vi "faux_daq.vi"() -> ()   [LabVIEW 2022 SP3]
panel:
  out "input_history":cluster{"Request":string, "Payload":variant}[](array[cluster])
  in  "clear_error":bool
  out "last output":T1
  in  "done":bool
  in  "payload":string caption="Request Payload"
  in  "request":string(combo) caption="Select Request"
  in  "send_request":bool
  in  "select_module":string(combo)="motion" caption="Select Test Module"
  out "output_history":T2(array[cluster])
  out "error out":errorcluster
  in  "error in":errorcluster
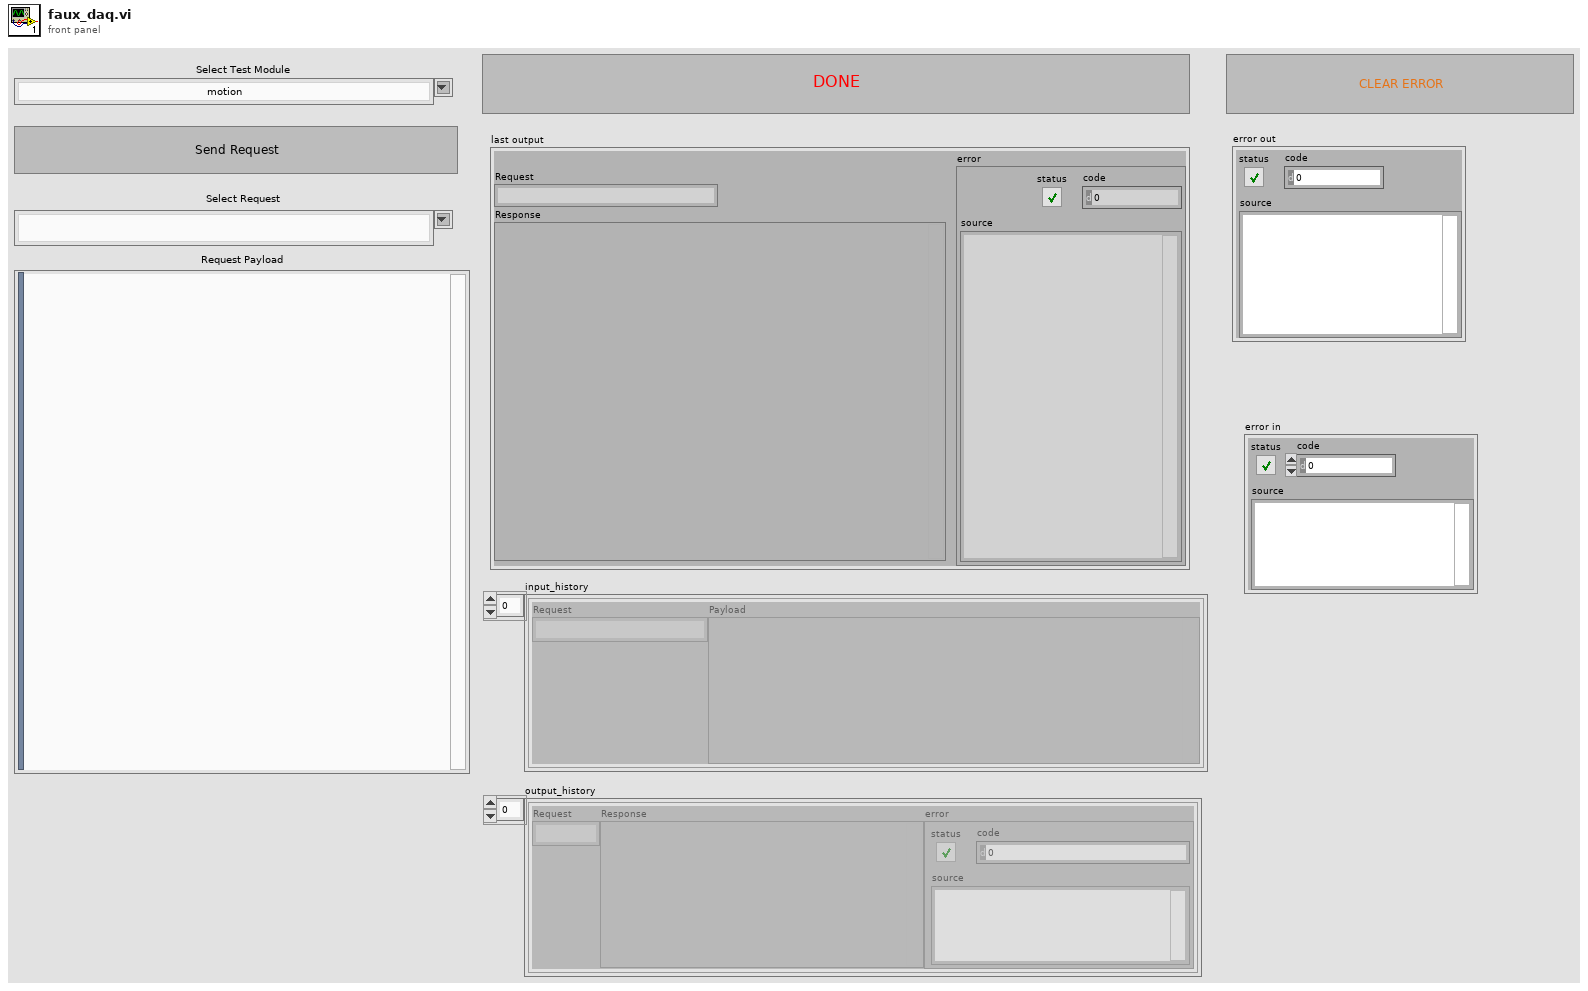
[diagram p1: front panel]
types:
  T1 = cluster{"Request":string, "Response":variant, "error":errorcluster}
  T2 = cluster{"Request":string, "Response":variant, "error":errorcluster}[]
  T3 = cluster{"request":string, "Response data":variant, "error IO":errorcluster}[]
  T4 = enum8{"Enabled", "Disabled", "Disabled and Grayed Out"}
  T5 = cluster{"request":string, "Response data":variant, "error IO":errorcluster}
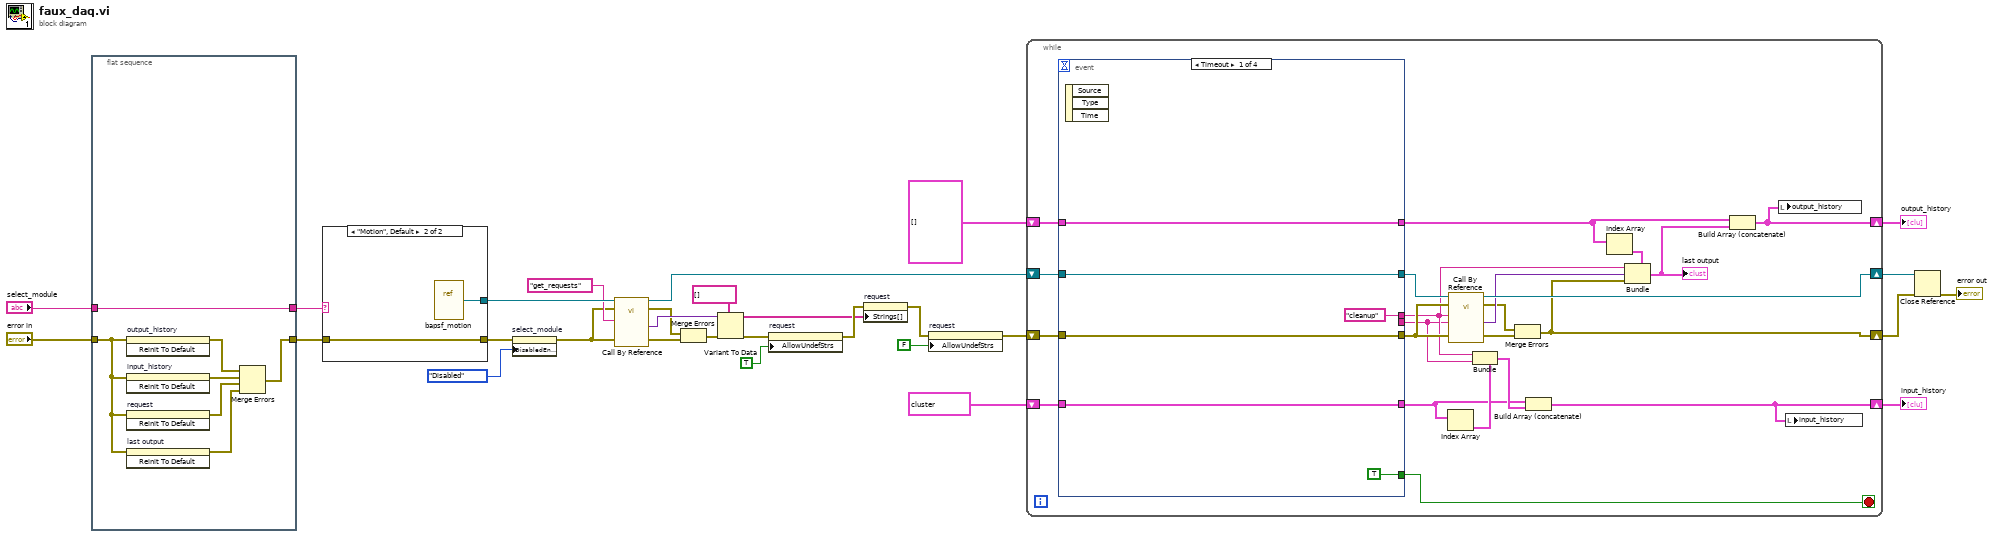
[diagram p0: block diagram]
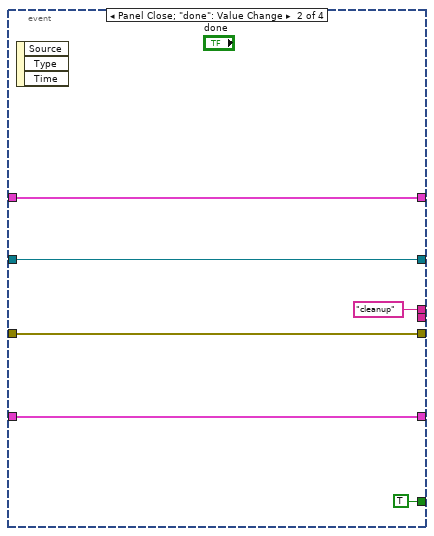
[diagram p2: hidden frame]
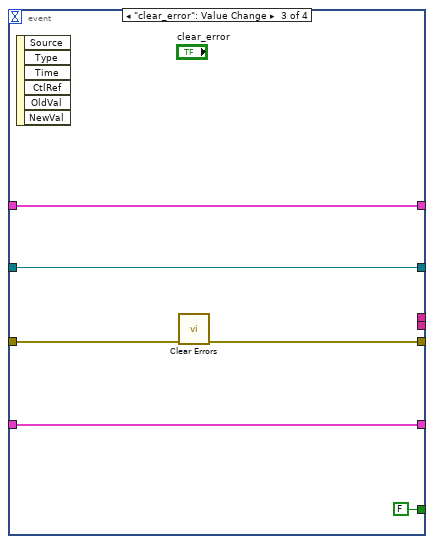
[diagram p3: hidden frame]
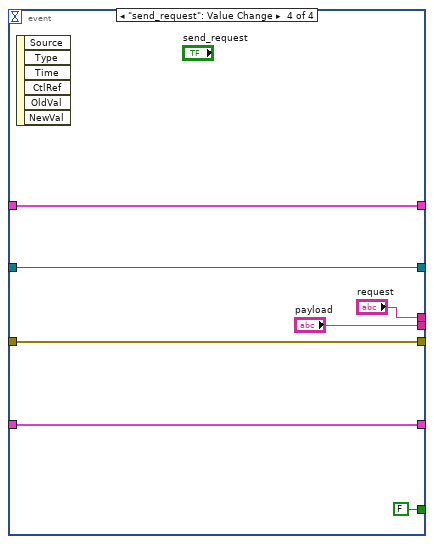
[diagram p4: hidden frame]
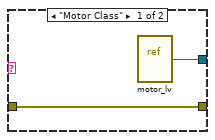
[diagram p5: hidden frame]
diagram:
  n1 = flat-sequence {
    tunnel: [w33] -> w29
    tunnel: "error in" -> [w35]
    tunnel: "select_module" -> [w36]
    tunnel: [w36] -> w5
    frame #0 {
      n2 = invoke on="output_history" class="Arr (strict)" method="Reinit To Default"(error in=w35) -> (error out=w34:errorcluster)  [unwired: 2 in, 2 out]
      n3 = invoke on="input_history" class="Arr (strict)" method="Reinit To Default"(error in=w35) -> (error out=w32:errorcluster)  [unwired: 2 in, 2 out]
      n4 = invoke on="request" class="CmbBox" method="Reinit To Default"(error in=w35) -> (error out=w31:errorcluster)  [unwired: 2 in, 2 out]
      n5 = invoke on="last output" class="Clust (strict)" method="Reinit To Default"(error in=w35) -> (error out=w30:errorcluster)  [unwired: 2 in, 2 out]
      n6 = Merge Errors(w34, w32, w31, w30) -> (w33:errorcluster)
    }
  }
  n7 = case shown="\"Motion\", Default" w5 {
    tunnel: w29 -> [w37 w39]
    tunnel: [w38 w40] -> w28
    tunnel: [w37 w39] -> w12
    frame "Motor Class" {
      n8 = vi-ref "motor_lv.vi"() -> (w38:refnum<vi>)
    }
    frame "Motion", Default {
      n9 = vi-ref "bapsf_motion.vi"() -> (w40:refnum<vi>)
    }
  }
  n10 = property on="select_module" class="CmbBox"(error in=w12, "DisabledEnum"=T4."Disabled" ("Disabled")) -> (error out=w11:errorcluster)  [unwired: 1 in, 1 out]
  n11 = call-by-ref "?"(reference=w28, error in=w11, "error in"=w11, "Request"="get_requests") -> (reference out=w15:refnum<vi>, error out=w18:errorcluster, 0:"error out"=w16:errorcluster, "Response data"=w26:variant)  [unwired: 4 in]
  n12 = Merge Errors(w18, w16) -> (w17:errorcluster)
  n13 = Variant To Data(error in=w17, type=string[] [], Variant=w26) -> (data=w21:string[], error out=w23:errorcluster)
  n14 = property on="request" class="CmbBox"(error in=w23, "AllowUndefStrs"=TRUE ("Allow Undefined Strings")) -> (error out=w22:errorcluster)  [unwired: 1 in, 1 out]
  n15 = property on="request" class="CmbBox"(error in=w22, "Strings[]"=w21) -> (error out=w20:errorcluster)  [unwired: 1 in, 1 out]
  n16 = property on="request" class="CmbBox"(error in=w20, "AllowUndefStrs"=FALSE ("Allow Undefined Strings")) -> (error out=w14:errorcluster)  [unwired: 1 in, 1 out]
  n17 = while {
    shift-right: [w58] -> w10
    shift-left: w15 -> [w60]
    shift-right: [w49] -> w9
    shift-left: w14 -> [w62]
    shift-right: [w48] -> w3
    shift-left: T3 [] -> [w56]
    shift-right: [w41] -> w1
    shift-left: cluster{"Request":string, "Payload":variant}[] [{"Request"="initialize", "Payload"=variant}, {"Request"="cleanup", "Payload"=variant}] ("input_history") -> [w47]
    stop <- w57 stop-if-true
    n18 = event shown="[0] Timeout" {
      selector: _ -> [_ _ _ _]
      dyn-events: _ -> [_ _ _ _]
      timeout: _ -> [_ _ _ _]
      tunnel: w62 -> [w68 w74 w78 w81]
      tunnel: [w68 w74 w77 w81] -> w61
      tunnel: w60 -> [w67 w70 w79 w83]
      tunnel: [w67 w70 w79 w83] -> w59
      tunnel: [TRUE TRUE FALSE FALSE] -> w57
      tunnel: ["cleanup" "cleanup" _ "request"] -> w45
      tunnel: w56 -> [w64 w71 w80 w87]
      tunnel: [w64 w71 w80 w87] -> w55
      tunnel: [_ _ _ "payload"] -> w44
      tunnel: w47 -> [w63 w69 w75 w82]
      tunnel: [w63 w69 w75 w82] -> w42
      event Timeout {
        n19 = event-data() -> ()  [unwired: 1 in, 3 out]
      }
      event Panel Close; "done": Value Change {
        n20 = event-data() -> ()  [unwired: 1 in, 3 out]
      }
      event "clear_error": Value Change {
        n21 = event-data() -> ()  [unwired: 1 in, 6 out]
        n22 = call <vilib>:"Clear Errors.vi"("error in (no error)"=w78) -> ("error out"=w77:errorcluster)  [unwired: 5 in, 1 out]
      }
      event "send_request": Value Change {
        n23 = event-data() -> ()  [unwired: 1 in, 6 out]
      }
    }
    n24 = Index Array(array=w42) -> (element=w46:cluster{"Request":string, "Payload":variant})  [unwired: 1 in]
    n25 = call-by-ref "?"(reference=w59, error in=w61, "error in"=w61, "Request data"=w44, "Request"=w45) -> (reference out=w58:refnum<vi>, error out=w51:errorcluster, 0:"error out"=w50:errorcluster, "Response data"=w52:variant)  [unwired: 3 in]
    n26 = Bundle(cluster=w46, "Request"=w45, "Payload"=w44) -> (w43:cluster{"Request":string, "Payload":variant})
    n27 = Merge Errors(w51, w50) -> (w49:errorcluster)
    n28 = Build Array (concatenate)(w42, w43) -> (w41:cluster{"Request":string, "Payload":variant}[])
    n29 = Index Array(array=w55) -> (element=w54:T5)  [unwired: 1 in]
    n30 = Bundle(cluster=w54, "request"=w45, "Response data"=w52, "error IO"=w49) -> (w53:T5)
    "last output" <- w53
    n31 = Build Array (concatenate)(w55, w53) -> (w48:T3)
    n32 = local write "output_history"(w48) -> ()
    n33 = local write "input_history"(w41) -> ()
  }
  "output_history" <- w3
  "input_history" <- w1
  n34 = Close Reference(reference=w10, error in (no error)=w9) -> (error out=→"error out":errorcluster)
